vi "Cleanup.vi"(8 "error in (no error)":errorcluster, 11 "ErrorManager in":refnum<class "ErrorManager.lvclass">) -> (0 "error out":errorcluster, 3 "ErrorManager out":refnum<class "ErrorManager.lvclass">)   [LabVIEW 2020, in "ErrorManager.lvlib" / "ErrorManager.lvclass"]
uses:
  ErrorManager.lvclass
  ErrorManager.lvclass/ErrorManager.ctl
  ErrorInfo.ctl
  ErrorType.ctl
  LabVIEWObjectInterfaces/IErrorManager/IErrorManager.lvclass
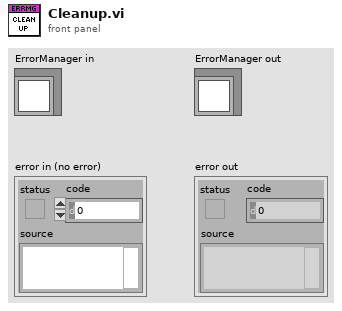
[diagram p1: front panel]
types:
  T1 = typedef "ErrorManager.lvlib/ErrorManager.lvclass/ErrorInfo.ctl" = cluster{"Time Stamp":timestamp, "Message":string, "Type":T2}
  T2 = typedef "LabVIEWObjectInterfaces.lvlib/IErrorManager.lvclass/ErrorType.ctl" = enum16{"Info", "Warning", "Error"}
  T3 = typedef "ErrorManager.lvlib/ErrorManager.lvclass/ErrorInfoArrayRef.ctl" = refnum<data-value>
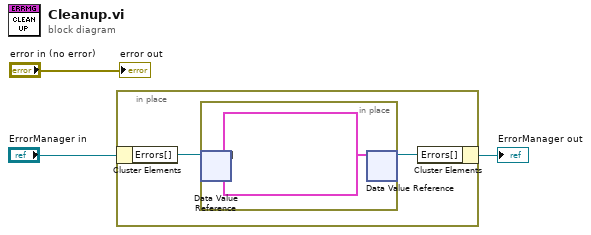
[diagram p0: block diagram]
diagram:
  n1 = in-place {
    n2 = in-place-cluster #1("ErrorManager in") -> ("Errors[]"=w5:T3)
    n3 = in-place {
      n4 = in-place-dvr #2(w5) -> ()  [unwired: 2 out]
      n5 = in-place-dvr #2(T1[] [] ("data value")) -> (w4:T3)  [unwired: 1 out]
    }
    n6 = in-place-cluster #1("Errors[]"=w4) -> (→"ErrorManager out":refnum<class "ErrorManager.lvclass">)
  }
  "error out" <- "error in (no error)"
